vi "Prepare stdin.vi"(8 "error in (no error)":errorcluster, 10 "BuildSpec Job Config":T1={"Project Path"=path "", "Build Name"="", "Target"="My Computer", "Clean"=FALSE, "Deploy"=FALSE}, 11 "Job.BuildSpec in":refnum<class "Job.BuildSpec.lvclass">) -> (0 "error out":errorcluster, 2 "Stdin":string, 3 "Job.BuildSpec out":refnum<class "Job.BuildSpec.lvclass">)   [LabVIEW 2013, in "Job.BuildSpec.lvclass"]
uses:
  Job.BuildSpec.lvclass
  BuildSpec Job Configuration -- cluster.ctl
  <vilib>/addons/_JKI.lib/Serialization/JSON/JKI JSON Serialization.lvlib
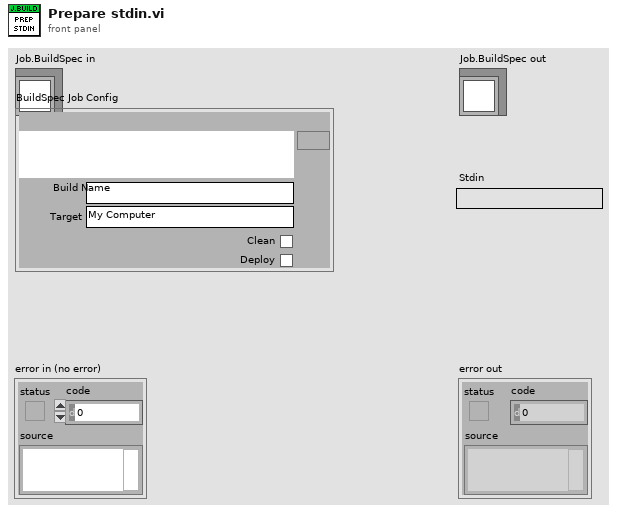
[diagram p1: front panel]
types:
  T1 = typedef "Job.BuildSpec.lvclass/BuildSpec Job Configuration -- cluster.ctl" = cluster{"Project Path":path, "Build Name":string, "Target":string, "Clean":bool, "Deploy":bool}
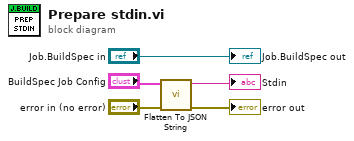
[diagram p0: block diagram]
diagram:
  n1 = call <vilib>:"Flatten To JSON String.vi"("error in (no error)"="error in (no error)", "Variant"="BuildSpec Job Config") -> ("error out"=→"error out":errorcluster, "JSON String"=→"Stdin":string)  [unwired: 8 in]
  "Job.BuildSpec out" <- "Job.BuildSpec in"
